vi "Setpoint.vi"(0 "VISA resource name":refnum<visa-resource-name>, 11 "error in (no error)":errorcluster) -> (4 "VISA resource name out":refnum<visa-resource-name>, 8 "Setpoint (0.00000E+0)":dbl min=0.0 max=100000000.0 step=1e-06 format="%^.5e", 15 "error out":errorcluster)   [LabVIEW 2020, in "Lake Shore Cryotronics 370.lvlib"]
doc: "This VI indicates the value of the temperature control setpoint."
uses:
  Lake Shore Cryotronics 370.lvlib
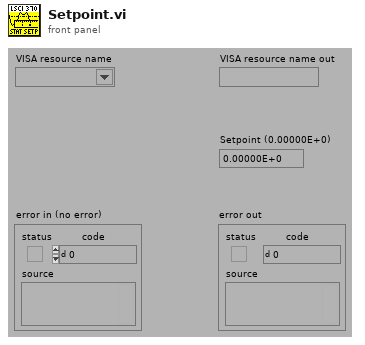
[diagram p1: front panel]
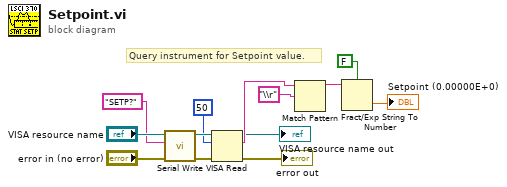
[diagram p0: block diagram]
diagram:
  # "Query instrument for Setpoint value."
  n1 = call "Serial Write.vi"("error in (no error)"="error in (no error)", "Write Buffer (\"\")"="SETP?", "VISA resource name"="VISA resource name") -> ("error out"=w11:errorcluster, "VISA resource name out"=w12:refnum<visa-resource-name>)  [unwired: 6 in, 1 out]
  n2 = VISA Read(VISA resource name=w12, byte count=50, error in (no error)=w11) -> (VISA resource name out=→"VISA resource name out":refnum<visa-resource-name>, read buffer=w9:string, error out=→"error out":errorcluster)  [unwired: 1 out]
  n3 = Match Pattern(string=w9, regular expression="\\r") -> (before substring=w13:string)  [unwired: 1 in, 3 out]
  n4 = Fract/Exp String To Number(use system decimal point (T)=FALSE, string=w13) -> (number=→"Setpoint (0.00000E+0)":dbl)  [unwired: 2 in, 1 out]
